vi "Destroy String List.vi"(8 "error in (no error)":errorcluster, 11 "StringList Reference":refnum<data-value>) -> (0 "error out":errorcluster, 2 "Final Items":string[](array[string]))   [LabVIEW 2015, in "StringList.lvlib" / "StringList.lvclass"]
uses:
  StringList.lvclass
  StringList.lvclass/StringList.ctl
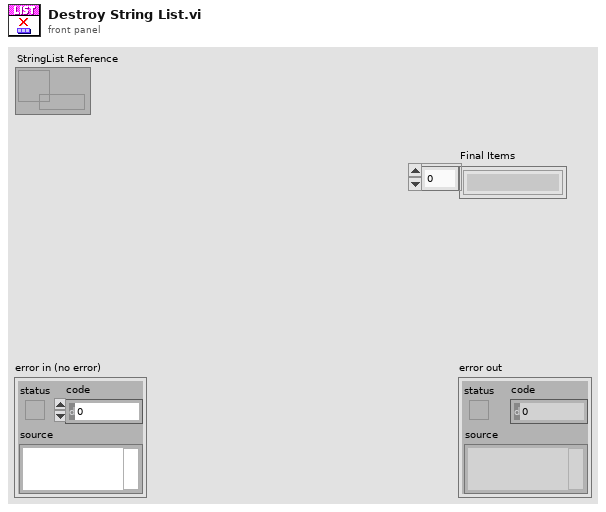
[diagram p1: front panel]
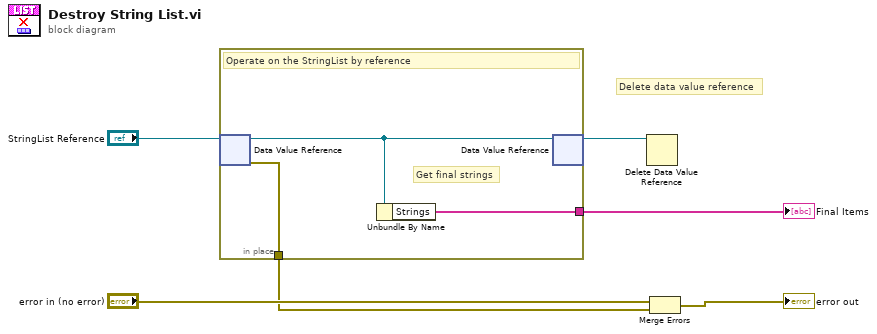
[diagram p0: block diagram]
diagram:
  # "Delete data value reference"
  n1 = in-place {
    in-place-border: [w9] -> w1
    in-place-border: [w7] -> w3
    # "Get final strings"
    # "Operate on the StringList by reference"
    n2 = in-place-dvr #1("StringList Reference") -> (w8:refnum<class "StringList.lvclass">, w9:errorcluster)
    n3 = Unbundle By Name(w8) -> ("Strings"=w7:string[])
    n4 = in-place-dvr #1(w8) -> (w2:refnum<data-value>)  [unwired: 1 out]
  }
  "Final Items" <- w3
  n5 = Delete Data Value Reference(data value reference=w2) -> ()  [unwired: 1 in, 2 out]
  n6 = Merge Errors("error in (no error)", w1) -> (→"error out":errorcluster)
